vi "write eight floats to csv line and file.vi"(0 "Path":path, 1 "item 3":dbl, 2 "item 2":dbl, 3 "item 1":dbl, 5 "item 4":dbl, 7 "item 5":dbl, 9 "item 6":dbl, 11 "error in (no error)":errorcluster, 12 "item 7":dbl, 13 "item 8":dbl) -> (4 "csv string":string, 15 "error out":errorcluster)   [LabVIEW 2013]
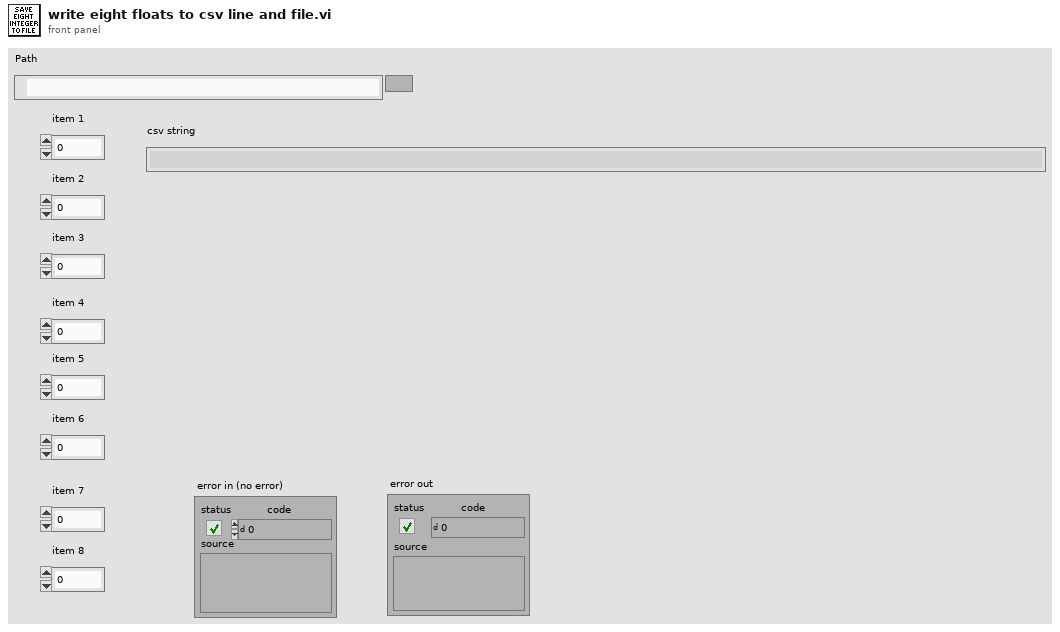
[diagram p1: front panel]
types:
  T1 = enum16{"open", "replace", "create", "open or create", "replace or create", "replace or create with confirmation"}
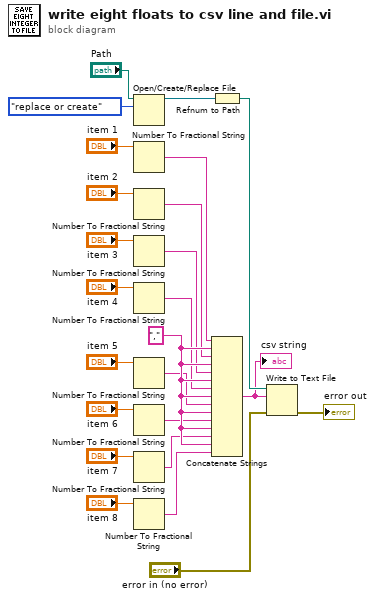
[diagram p0: block diagram]
diagram:
  w21 = "," ("element")
  n1 = Open/Create/Replace File(file path (use dialog)="Path", operation (0:open)=T1."replace or create") -> (refnum out=w24:refnum<file>)  [unwired: 4 in, 2 out]
  n2 = Number To Fractional String(number="item 1") -> (F-format string=w8:string)  [unwired: 3 in]
  n3 = Number To Fractional String(number="item 2") -> (F-format string=w7:string)  [unwired: 3 in]
  n4 = Number To Fractional String(number="item 3") -> (F-format string=w6:string)  [unwired: 3 in]
  n5 = Number To Fractional String(number="item 4") -> (F-format string=w5:string)  [unwired: 3 in]
  n6 = Number To Fractional String(number="item 5") -> (F-format string=w4:string)  [unwired: 3 in]
  n7 = Number To Fractional String(number="item 6") -> (F-format string=w3:string)  [unwired: 3 in]
  n8 = Number To Fractional String(number="item 7") -> (F-format string=w2:string)  [unwired: 3 in]
  n9 = Number To Fractional String(number="item 8") -> (F-format string=w1:string)  [unwired: 3 in]
  n10 = Refnum to Path(1:w24) -> (0:w20:path)
  n11 = Concatenate Strings(w8, w21, w7, w21, w6, w21, w5, w21, w4, w21, w3, w21, w2, w21, w1) -> (w19:string)
  "csv string" <- w19
  n12 = Write to Text File(file (use dialog)=w20, text=w19, error in="error in (no error)") -> (error out=→"error out":errorcluster)  [unwired: 1 in, 2 out]
